vi "Server Generate ACK Event.vi"(6 "error data to send (in error case)":errorcluster, 8 "error in":errorcluster, 9 "ACK (True)":bool=TRUE, 10 "header":string, 11 "server event ref":refnum<vi>) -> (0 "error out":errorcluster)   [LabVIEW 2013]
doc: "Sends simple ACK no ACK answer event to server. If 'error data to send' contains error, it will send it as error message ignoring ACK state."
uses:
  octave/infolib.lvlibp/Private/Add matrix polymorph parts/1D String.vi
  octave/infolib.lvlibp
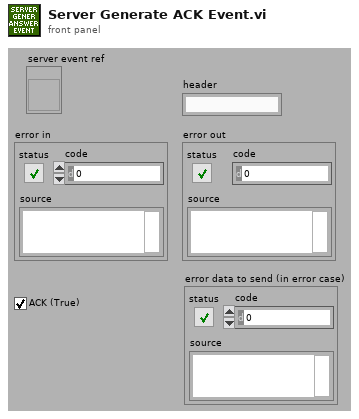
[diagram p1: front panel]
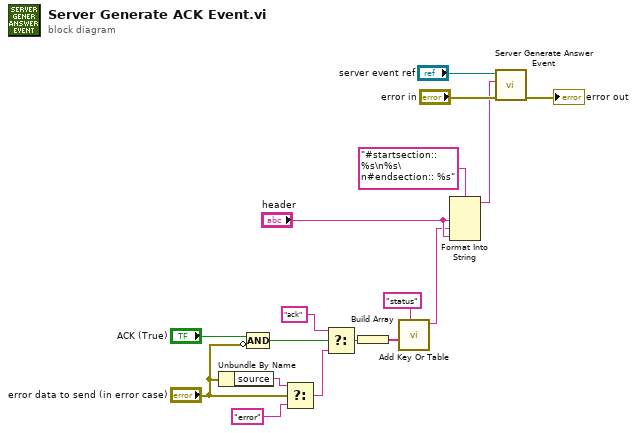
[diagram p0: block diagram]
diagram:
  n1 = Unbundle By Name("error data to send (in error case)") -> ("source"=w10:string)
  n2 = Compound Arithmetic op=AND("ACK (True)", invert "error data to send (in error case)") -> (w7:bool)
  n3 = Select(t=w10, s="error data to send (in error case)", f="error") -> (s? t:f=w8:string)
  n4 = Select(t="ack", s=w7, f=w8) -> (s? t:f=w2:string)
  n5 = Build Array(w2) -> (w3:string[])
  n6 = call-poly "Add Key Or Table.vi"("key description"="status", "string"=w3) -> ("info data out"=w1:string)  [unwired: 8 in, 1 out]
  n7 = Format Into String(format string="#startsection:: %s\n%s\n#endsection:: %s", "header", w1, "header") -> (resulting string=w11:string)  [unwired: 2 in, 1 out]
  n8 = call "Server Generate Answer Event.vi"("error in"="error in", "event data"=w11, "server event ref"="server event ref") -> ("error out"=→"error out":errorcluster)  [unwired: 8 in]
